vi "Find Library in Project.vi"(8 "error in":errorcluster, 9 "DQMH Modules Refs":refnum<vi>[](array[refnum]), 10 "Project Ref":refnum<vi>, 11 "DQMH Lib Ref":refnum<vi>) -> (0 "error out":errorcluster)   [LabVIEW 2019]
uses:
  Panther Dashboard.lvlib
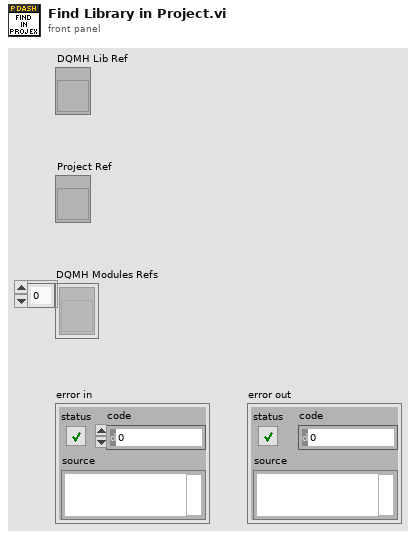
[diagram p1: front panel]
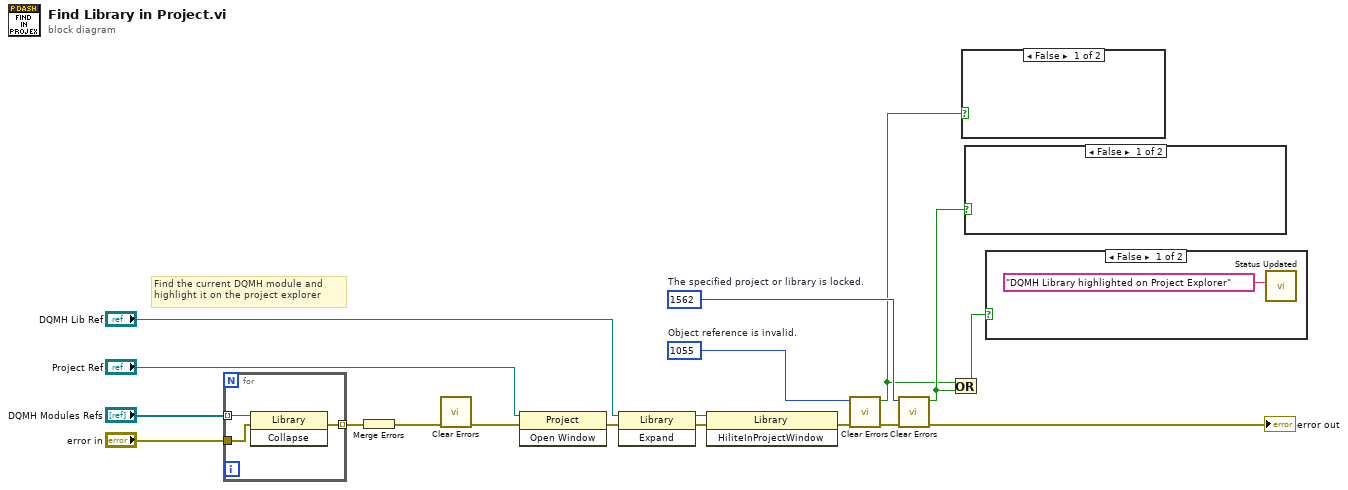
[diagram p0: block diagram]
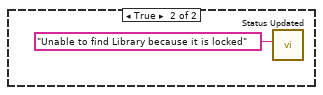
[diagram p3: hidden frame]
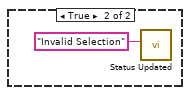
[diagram p4: hidden frame]
diagram:
  w5 = 1562  # The specified project or library is locked.
  w9 = 1055  # Object reference is invalid.
  # "Find the current DQMH module and\nhighlight it on the project explorer"
  n1 = for {
    tunnel: "DQMH Modules Refs" -> [w19] mode=indexing
    tunnel: [w21] -> w11 mode=indexing
    tunnel: "error in" -> [w20]
    n2 = invoke class="Library" method="Collapse"(reference=w19, error in=w20) -> (error out=w21:errorcluster)  [unwired: 1 in, 2 out]
  }
  n3 = Merge Errors(w11) -> (w17:errorcluster)
  n4 = call <vilib>:"Clear Errors.vi"("error in (no error)"=w17) -> ("error out"=w1:errorcluster)  [unwired: 5 in, 1 out]
  n5 = invoke class="Project" method="Open Window"(reference="Project Ref", error in=w1) -> (error out=w16:errorcluster)  [unwired: 1 in, 2 out]
  n6 = invoke class="Library" method="Expand"(reference="DQMH Lib Ref", error in=w16) -> (reference out=w10:refnum<vi>, error out=w15:errorcluster)  [unwired: 1 in, 1 out]
  n7 = invoke class="Library" method="HiliteInProjectWindow"(reference=w10, error in=w15) -> (error out=w18:errorcluster)  [unwired: 1 in, 2 out]
  n8 = call <vilib>:"Clear Errors.vi"("error in (no error)"=w18, "specific error code to clear (0: all)"=w9) -> ("error out"=w14:errorcluster, "specific error cleared?"=w3:bool)  [unwired: 4 in]
  n9 = call <vilib>:"Clear Errors.vi"("error in (no error)"=w14, "specific error code to clear (0: all)"=w5) -> ("error out"=→"error out":errorcluster, "specific error cleared?"=w4:bool)  [unwired: 4 in]
  n10 = Or(x=w3, y=w4) -> (x .or. y?=w2:bool)
  n11 = case shown="False" w3 {
    frame False {
    }
    frame True {
      n12 = call "Status Updated.vi"("Status"="Invalid Selection") -> ()  [unwired: 10 in, 1 out]
    }
  }
  n13 = case shown="False" w4 {
    frame False {
    }
    frame True {
      n14 = call "Status Updated.vi"("Status"="Unable to find Library because it is locked") -> ()  [unwired: 10 in, 1 out]
    }
  }
  n15 = case shown="False" w2 {
    frame False {
      n16 = call "Status Updated.vi"("Status"="DQMH Library highlighted on Project Explorer") -> ()  [unwired: 10 in, 1 out]
    }
    frame True {
    }
  }
